vi "dfd_Rotate FIR Transposed.vi"(5 "#taps per phase":i32, 9 "state idx":T1={"start"=0, "stepsize"=1}, 10 "state in":i64[](array[numeric])) -> (2 "state out":i64[](array[numeric]), 3 "y":i64)   [LabVIEW 2017, in "NI_DigFilter_FXP.lvlib"]
uses:
  <vilib>/addons/Digital Filter Design/NI_DigFilter_FXP.lvlib
  <vilib>/addons/Digital Filter Design/_Objects.llb/dfd_Index Config.ctl
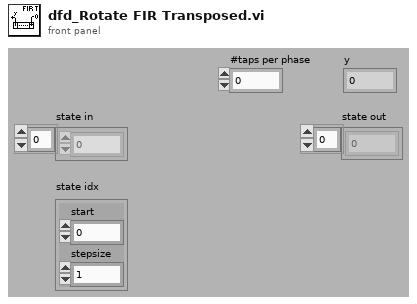
[diagram p1: front panel]
types:
  T1 = typedef "dfd_Index Config.ctl" = cluster{"start":i32, "stepsize":i32}
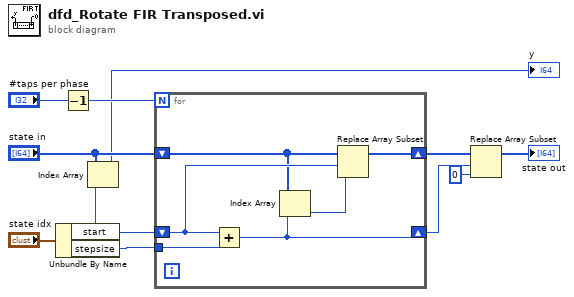
[diagram p0: block diagram]
diagram:
  n1 = Unbundle By Name("state idx") -> ("start"=w6:i32, "stepsize"=w5:i32)
  n2 = Decrement(x="#taps per phase") -> (x-1=w10:i32)
  n3 = Index Array(array="state in", index=w6) -> (element=→"y":i64)
  n4 = for {
    N: w10 -> [_]
    shift-right: [w12] -> w4
    shift-left: "state in" -> [w15]
    shift-right: [w14] -> w3
    shift-left: w6 -> [w16]
    tunnel: w5 -> [w17]
    n5 = Add(x=w16, y=w17) -> (x+y=w14:i32)
    n6 = Index Array(array=w15, index=w14) -> (element=w13:i64)
    n7 = Replace Array Subset(array=w15, new element=w13, index=w16) -> (w12:i64[])
  }
  n8 = Replace Array Subset(array=w4, new element=i64 0 ("new element/subarray"), index=w3) -> (→"state out":i64[])
